vi "bit conversion.vi"() -> ()   [LabVIEW 2013]
uses:
  <vilib>/NI/Tools/String/Tools_String.lvlib
panel:
  out "token array":string[](array[string])
  out "*(type *) &x":string
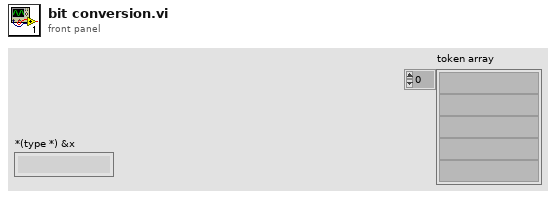
[diagram p1: front panel]
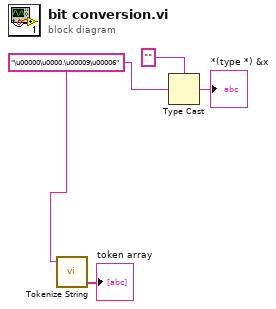
[diagram p0: block diagram]
diagram:
  w1 = "\u00000\u0000.\u00009\u00006"
  n1 = call <vilib>:"Tokenize String.vi"("input string"=w1) -> ("token array"=→"token array":string[])  [unwired: 3 in, 1 out]
  n2 = Type Cast(type="", x=w1) -> (*(type *) &x=→"*(type *) &x":string)
